vi "Set Data.vi"(0 "1D Waveform Data in":refnum<class "1D Waveform Logging Data.lvclass">, 5 "Group Name":string, 7 "Channel Names":string[](array[string]), 9 "Data":waveform(dbl)[](array[waveform]), 11 "error in (no error)":errorcluster) -> (4 "1D Waveform Data out":refnum<class "1D Waveform Logging Data.lvclass">, 15 "error out":errorcluster)   [LabVIEW 2024, in "Logging Data.lvlib" / "1D Waveform Logging Data.lvclass"]
uses:
  1D Waveform Logging Data.lvclass
  C:/Users/uspoaotto/OneDrive - Oregon Tool/Desktop/working copies/dataLogger/Logging Data/Logging Data/Logging Data.lvclass
  1D Waveform Logging Data.lvclass/1D Waveform Logging Data.ctl
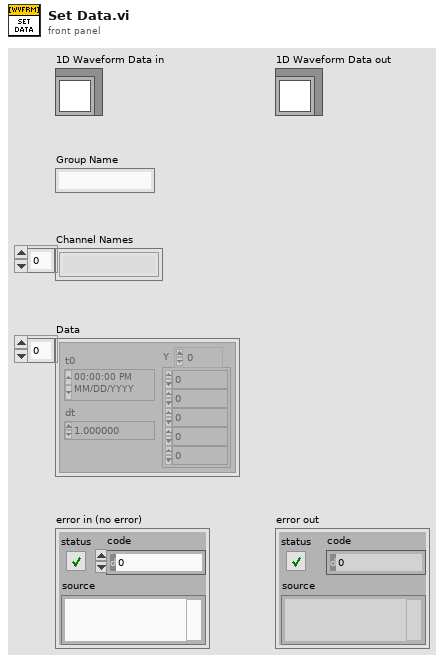
[diagram p1: front panel]
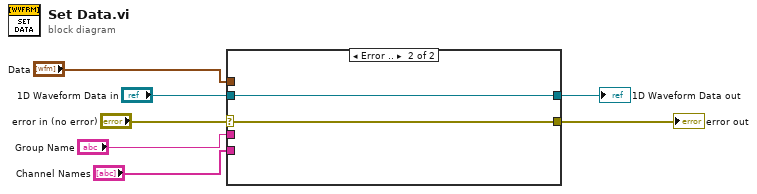
[diagram p0: block diagram]
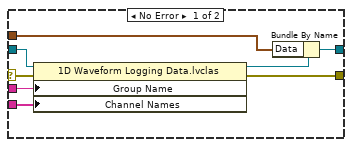
[diagram p2: hidden frame]
diagram:
  n1 = case shown="Error .." "error in (no error)" {
    selector: "error in (no error)" -> [w9 w17]
    tunnel: "1D Waveform Data in" -> [w15 w16]
    tunnel: "Data" -> [w13 _]
    tunnel: "Group Name" -> [w12 _]
    tunnel: "Channel Names" -> [w11 _]
    tunnel: [w10 w16] -> w3
    tunnel: [w8 w17] -> w1
    frame No Error {
      n2 = property class="1D Waveform Logging Data.lvclas"(reference=w15, error in=w9, "Group Name"=w12, "Channel Names"=w11) -> (reference out=w14:refnum<class "1D Waveform Logging Data.lvclass">, error out=w8:errorcluster)
      n3 = Bundle By Name(cluster=w14, "Data"=w13) -> (w10:refnum<class "1D Waveform Logging Data.lvclass">)
    }
    frame Error {
    }
  }
  "1D Waveform Data out" <- w3
  "error out" <- w1
